vi "Set Persistent Mode.vi"(8 "error in (no error)":errorcluster, 11 "Instrument.Oxford1820 in":refnum<class "Instrument.Oxford1820.lvclass">) -> (0 "error out":errorcluster, 3 "Instrument.Oxford1820 out":refnum<class "Instrument.Oxford1820.lvclass">)   [LabVIEW 2016, in "Instrument.Oxford1820.lvclass"]
uses:
  Instrument.Oxford1820.lvclass
  <instrlib>/Mercury iXX/Public/Libraries/Magnet/Controls/Switch Heater.ctl
  <instrlib>/Mercury iXX/Public/Libraries/Magnet.lvlib
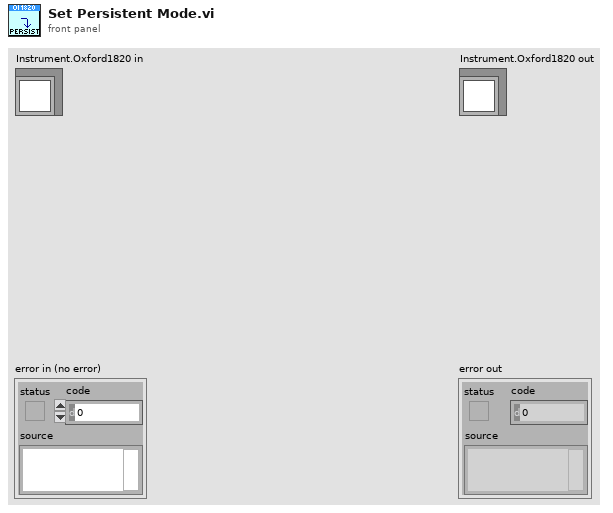
[diagram p1: front panel]
types:
  T1 = typedef "Mercury iXX.lvlib/Magnet.lvlib/Switch Heater.ctl" = string
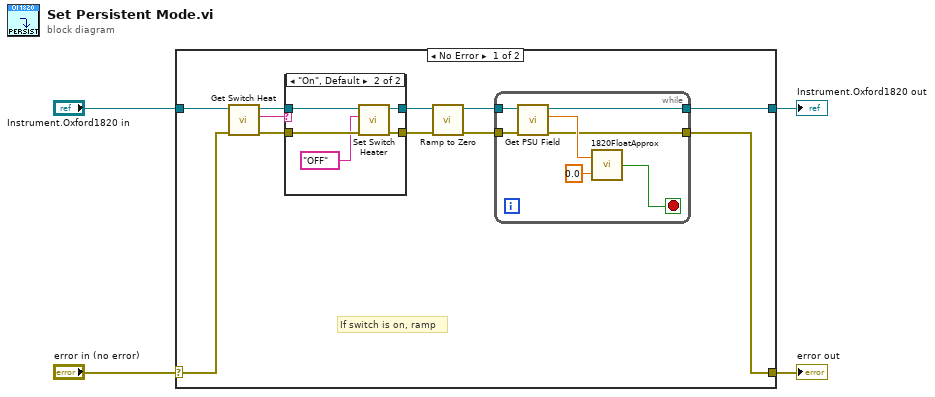
[diagram p0: block diagram]
diagram:
  n1 = case shown="No Error" "error in (no error)" {
    selector: "error in (no error)" -> [w12 w31]
    tunnel: [w10 w31] -> w3
    tunnel: [w13 w30] -> w1
    tunnel: "Instrument.Oxford1820 in" -> [w15 w30]
    frame No Error {
      # "If switch is on, ramp"
      n2 = call-dynamic "Get Switch Heat.vi"("error in (no error)"=w12, "Instrument.Oxford1820 in"=w15) -> ("error out"=w11:errorcluster, "Switch Heater Status"=w5:string, "Instrument.Oxford1820 out"=w14:refnum<class "Instrument.Oxford1820.lvclass">)  [unwired: 6 in, 1 out]
      n3 = case shown="\"On\", Default" w5 {
        tunnel: w14 -> [w17 w22]
        tunnel: w11 -> [w16 w21]
        tunnel: [w17 w20] -> w7
        tunnel: [w16 w19] -> w6
        frame "Off" {
        }
        frame "On", Default {
          n4 = call-dynamic "Set Switch Heater.vi"("error in (no error)"=w21, "Switch Heater"=T1 "OFF", "Instrument.Oxford1820 in"=w22) -> ("error out"=w19:errorcluster, "Instrument.Oxford1820 out"=w20:refnum<class "Instrument.Oxford1820.lvclass">)  [unwired: 7 in]
        }
      }
      n5 = call-dynamic "Ramp to Zero.vi"("error in (no error)"=w6, "Instrument.Oxford1820 in"=w7) -> ("error out"=w9:errorcluster, "Instrument.Oxford1820 out"=w8:refnum<class "Instrument.Oxford1820.lvclass">)  [unwired: 8 in]
      n6 = while {
        tunnel: w9 -> [w29]
        tunnel: w8 -> [w28]
        tunnel: [w24] -> w10
        tunnel: [w23] -> w13
        stop <- w25 stop-if-true
        n7 = call-dynamic "Get PSU Field.vi"("error in (no error)"=w29, "Instrument.Oxford1820 in"=w28) -> ("error out"=w24:errorcluster, "PSU Field (T)"=w27:dbl, "Instrument.Oxford1820 out"=w23:refnum<class "Instrument.Oxford1820.lvclass">)  [unwired: 7 in]
        n8 = call "1820FloatApprox.vi"("y"=0.0, "x"=w27) -> ("x ~ y?"=w25:bool)
      }
    }
    frame Error {
    }
  }
  "error out" <- w3
  "Instrument.Oxford1820 out" <- w1
